vi "I2C_WriteMasterACK_2.vi"(6 "ACK":bool, 8 "error in":errorcluster, 10 "HalfCycle(Ticks)":u32, 11 "InterByteTransmitDelay(Ticks)":u32) -> (0 "error out":errorcluster, 2 "Status":i16)   [LabVIEW 2019]
doc: "Writes the Master ACK in response to a Byte of data being received from the Slave Device.\n\nVI Written By:\nPeter Fuller\nSenior Engineer\nplf Consulting, LLC\n617.699.2201"
uses:
  <vilib>/eio/EIONode/EIONode.xnode
  Instance           1 26Saved   I2C_WriteMasterACK .vi
  Instance           2 26Saved   I2C_WriteMasterACK .vi
  Instance           3 26Saved   I2C_WriteMasterACK .vi
  <vilib>/eio/EIOMethodNode/EIOMethodNode.xnode
  <vilib>/rvi/eio/common/nirviEmuTemplateMethod_errors.vi
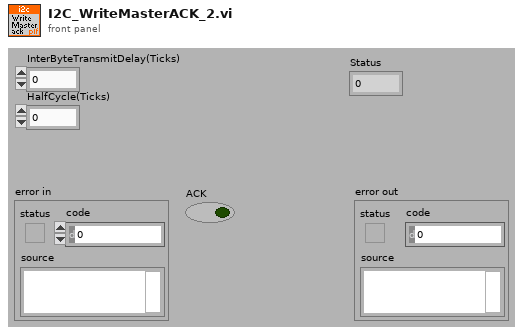
[diagram p1: front panel]
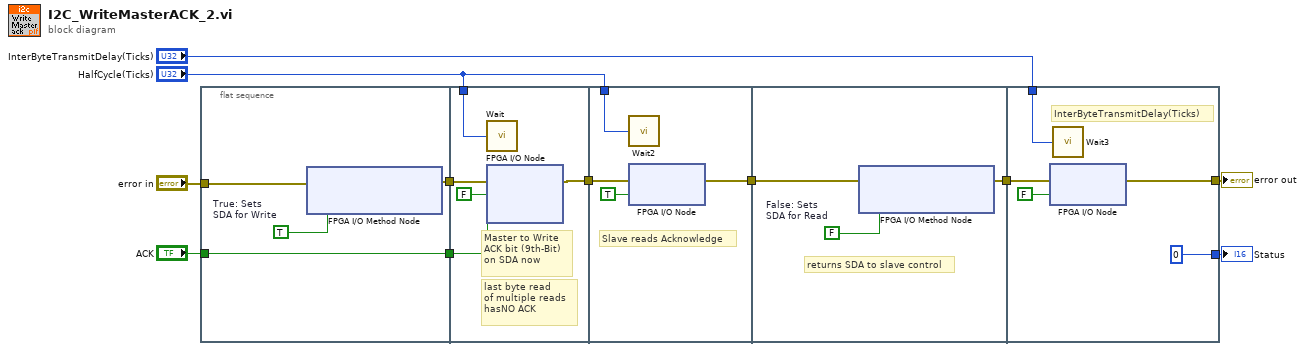
[diagram p0: block diagram]
diagram:
  n1 = flat-sequence {
    tunnel: "error in" -> [w14]
    tunnel: "ACK" -> [w15]
    tunnel: [w15] -> w9
    tunnel: [w12] -> w8
    tunnel: [w18] -> w7
    tunnel: w9 -> [w16]
    tunnel: w8 -> [w19]
    tunnel: "HalfCycle(Ticks)" -> [w17]
    tunnel: w7 -> [w23]
    tunnel: "HalfCycle(Ticks)" -> [w22]
    tunnel: [w21] -> w4
    tunnel: [w26] -> w3
    tunnel: w4 -> [w25]
    tunnel: w3 -> [w31]
    tunnel: "InterByteTransmitDelay(Ticks)" -> [w29]
    tunnel: [w30] -> w5
    tunnel: [i16 0] -> w1
    frame #0 {
      w13 = TRUE  # True: Sets  SDA for Write
      n2 = xnode "FPGA I/O Method Node"("error in"=w14, "Enable"=w13) -> ("error out"=w12:errorcluster)  [unwired: 1 in, 1 out]
    }
    frame #1 {
      # "last byte read \nof multiple reads \nhasNO ACK"
      # "Master to Write\nACK bit (9th-Bit)\non SDA now"
      n3 = call "Wait"("Count(Ticks)"=w17) -> ()  [unwired: 1 out]
      n4 = xnode "FPGA I/O Node"("error in"=w19, "SCL2"=FALSE ("Value"), "SDA2"=w16) -> ("error out"=w18:errorcluster)  [unwired: 2 in, 2 out]
    }
    frame #2 {
      # "Slave reads Acknowledge"
      n5 = call "Wait2"("Count(Ticks)"=w22) -> ()  [unwired: 1 out]
      n6 = xnode "FPGA I/O Node"("error in"=w23, "SCL2"=TRUE ("Value")) -> ("error out"=w21:errorcluster)  [unwired: 1 in, 1 out]
    }
    frame #3 {
      w27 = FALSE  # False: Sets  SDA for Read
      # "returns SDA to slave control"
      n7 = xnode "FPGA I/O Method Node"("error in"=w25, "Enable"=w27) -> ("error out"=w26:errorcluster)  [unwired: 1 in, 1 out]
    }
    frame #4 {
      # "InterByteTransmitDelay(Ticks)"
      n8 = xnode "FPGA I/O Node"("error in"=w31, "SCL2"=FALSE ("Value")) -> ("error out"=w30:errorcluster)  [unwired: 1 in, 1 out]
      n9 = call "Wait3"("Count(Ticks)"=w29) -> ()  [unwired: 1 out]
    }
  }
  "error out" <- w5
  "Status" <- w1
